vi "MH_SetInputChannels.vi"(10 "Channels new":T1[](array[typedef]) {"DeadTime" min=800 max=160000 step=1; "Edge" items=["falling", "rising"]; "Offset" min=-100000 max=100000 step=10; "Level" min=-1200 max=1200 step=1}, 11 "Channels old":T1[](array[typedef]) {"DeadTime" min=800 max=160000 step=1; "Edge" items=["falling", "rising"]; "Offset" min=-100000 max=100000 step=10; "Level" min=-1200 max=1200 step=1}) -> (2 "SetInpChan":T2[](array[typedef]), 3 "Channels":T1[](array[typedef]) {"DeadTime" min=800 max=160000 step=1; "Edge" items=["falling", "rising"]; "Offset" min=-100000 max=100000 step=10; "Level" min=-1200 max=1200 step=1})   [LabVIEW 2017]
uses:
  Types/MH_SetInpChanData.ctl
  Types/MH_SetInpChanCmds.ctl
  Types/MH_InputChannel.ctl
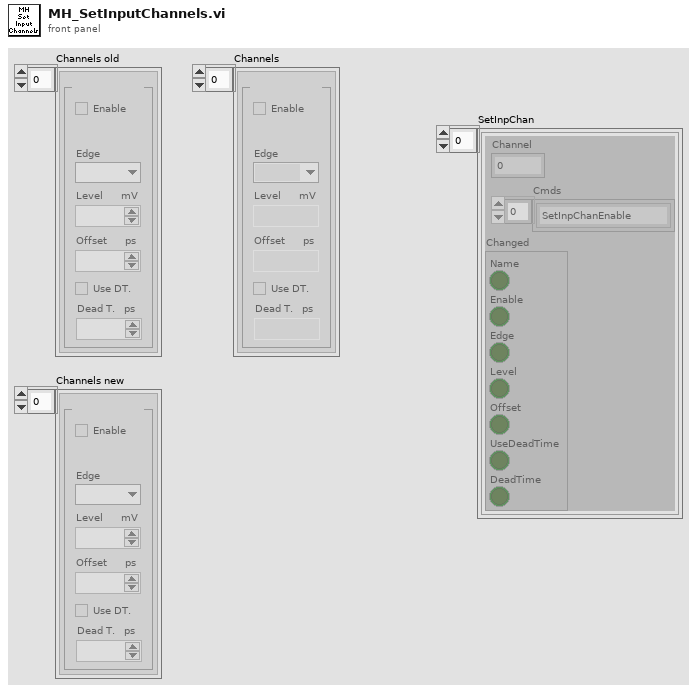
[diagram p1: front panel]
types:
  T1 = typedef "MH_InputChannel.ctl" = cluster{"Name":string, "Enable":bool, "Edge":i32, "Level":i32, "Offset":i32, "UseDeadTime":bool, "DeadTime":i32}
  T2 = typedef "MH_SetInpChanData.ctl" = cluster{"Channel":i32, "Cmds":T3[], "Changed":cluster{"Name":bool, "Enable":bool, "Edge":bool, "Level":bool, "Offset":bool, "UseDeadTime":bool, "DeadTime":bool}}
  T3 = typedef "MH_SetInpChanCmds.ctl" = enum16{"SetInpChanEnable", "SetInpChanOffset", "SetInpChanDeadTime", "SetInpChanTrg"}
  T4 = cluster{"Name":bool, "Enable":bool, "Edge":bool, "Level":bool, "Offset":bool, "UseDeadTime":bool, "DeadTime":bool}[]
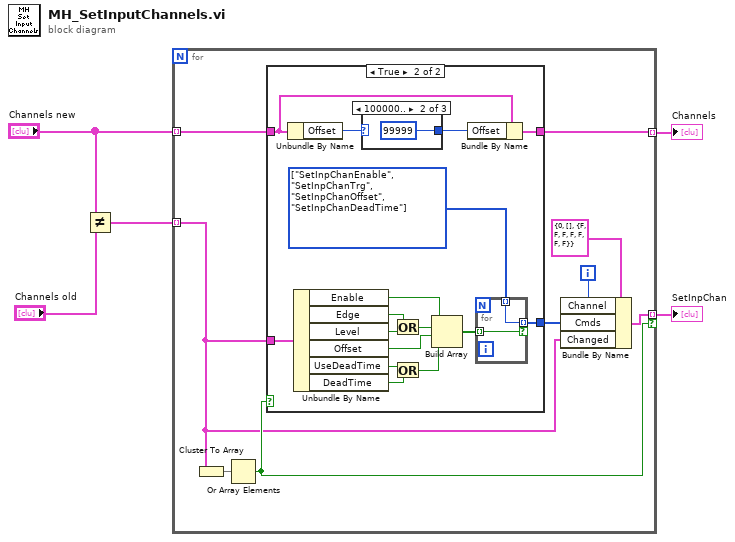
[diagram p0: block diagram]
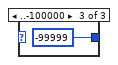
[diagram p4: hidden frame]
diagram:
  n1 = Not Equal?(x="Channels old", y="Channels new") -> (x != y?=w2:T4)
  n2 = for {
    tunnel: w2 -> [w6] mode=indexing
    tunnel: [w7] -> w5 mode=indexing if=w13
    tunnel: "Channels new" -> [w12] mode=indexing
    tunnel: [w11] -> w4 mode=indexing
    i -> [w9]
    n3 = Cluster To Array(cluster=w6) -> (array=w14:bool[])
    n4 = Or Array Elements(Boolean array=w14) -> (logical OR=w13:bool)
    n5 = case shown="True" w13 {
      tunnel: w6 -> [_ w31]
      tunnel: [_ w21] -> w8
      tunnel: w12 -> [w15 w19]
      tunnel: [w15 w17] -> w11
      frame False {
      }
      frame True {
        w16 = T3[] [enum."SetInpChanEnable", enum."SetInpChanTrg", enum."SetInpChanOffset", enum."SetInpChanDeadTime"] items=["SetInpChanEnable", "SetInpChanOffset", "SetInpChanDeadTime", "SetInpChanTrg"]
        n6 = Unbundle By Name(w19) -> ("Offset"=w20:i32)
        n7 = Unbundle By Name(w31) -> ("Enable"=w26:bool, "Edge"=w28:bool, "Level"=w27:bool, "Offset"=w24:bool, "UseDeadTime"=w29:bool, "DeadTime"=w30:bool)
        n8 = case shown="100000.." w20 {
          selector: w20 -> [w32 _ _]
          tunnel: [w32 99999 ("SyncOffset") -99999 ("SyncOffset")] -> w18
          frame Default {
          }
          frame 100000.. {
          }
          frame ..-100000 {
          }
        }
        n9 = Or(x=w28, y=w27) -> (x .or. y?=w25:bool)
        n10 = Or(x=w29, y=w30) -> (x .or. y?=w23:bool)
        n11 = Build Array(w26, w25, w24, w23) -> (w22:bool[])
        n12 = Bundle By Name(cluster=w19, "Offset"=w18) -> (w17:T1)
        n13 = for {
          tunnel: w22 -> [w35] mode=indexing
          tunnel: w16 -> [w36] mode=indexing
          tunnel: [w36] -> w21 mode=indexing if=w35
        }
      }
    }
    n14 = Bundle By Name(cluster=T2 {"Channel"=0, "Cmds"=[], "Changed"={"Name"=FALSE, "Enable"=FALSE, "Edge"=FALSE, "Level"=FALSE, "Offset"=FALSE, "UseDeadTime"=FALSE, "DeadTime"=FALSE}}, "Channel"=w9, "Cmds"=w8, "Changed"=w6) -> (w7:T2)
  }
  "SetInpChan" <- w5
  "Channels" <- w4
